vi "generate_pulse.vi"() -> ()   [LabVIEW 2018]
uses:
  Control 1.ctl
  <vilib>/DAQmx/write.llb/DAQmx Write (Analog 1D Wfm NChan NSamp).vi
  <vilib>/DAQmx/create/channels.llb/DAQmx Create Channel (AO-Voltage-Basic).vi
  <vilib>/DAQmx/configure/timing.llb/DAQmx Timing (Sample Clock).vi
  <vilib>/DAQmx/miscellaneous.llb/DAQmx Fill In Error Info.vi
  <resource>/objmgr/daqmx.rc
panel:
  in  "Exit":bool
  out "Actual Sample Rate 2":dbl=400000.0 format="%0.2f"
  in  "Physical Channel(s)":tag="Dev3/ao0:1"
  in  "Min Voltage 2":dbl=-10.0
  in  "Max Voltage 2":dbl=10.0
  in  "Sample Clock Source":tag="OnboardClock"
  in  "Sample Rate 2":dbl=400000.0 format="%#_6p"
  in  "Pulser Cycles":i32=10
  out "Sample per Channel AO":dbl=20000.0
  in  "Tab Control 4":enum32{"Basic", "Gaussian", "Chirp"}(tab)=enum."Chirp"
  in  "Pulse Basic":T2={"Basic amp"=1.5, "Duty cycle %"=50.0, "Basic freq (Hz)"=200, "Basic Type"=2} {"Basic Type" items=["Sine Wave", "Triangle Wave", "Square Wave", "Sawtooth Wave"]; "Duty cycle %" format="%#.2f"; "Basic amp" format="%0.2p"}
  in  "Pulse Gaussian":T3={"Gauss amp"=2.8, "Gauss Nor. Band"=0.5, "Gauss atten (dB)"=6.0, "Gauss freq (Hz)"=1000.0}
  in  "Pulse chirp":T4={"Chirp amp"=2.1, "Chirp f2"=1500.0, "Chirp f1"=500.0} {"Chirp f1" format="%0.2f"; "Chirp f2" format="%0.2f"; "Chirp amp" format="%0.2f"}
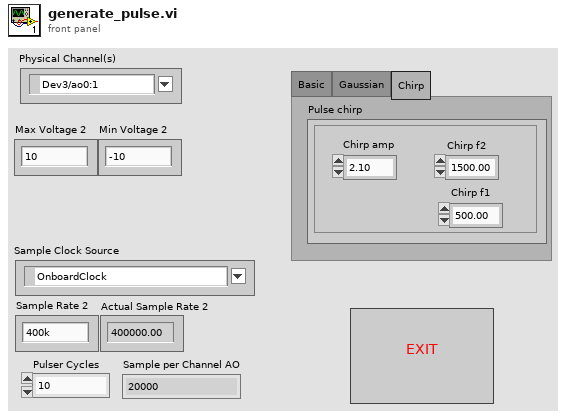
[diagram p1: front panel]
types:
  T1 = typedef "Control 1.ctl" = dbl
  T2 = cluster{"Basic amp":T1, "Duty cycle %":dbl, "Basic freq (Hz)":u16, "Basic Type":u16}
  T3 = cluster{"Gauss amp":dbl, "Gauss Nor. Band":dbl, "Gauss atten (dB)":dbl, "Gauss freq (Hz)":dbl}
  T4 = cluster{"Chirp amp":dbl, "Chirp f2":dbl, "Chirp f1":dbl}
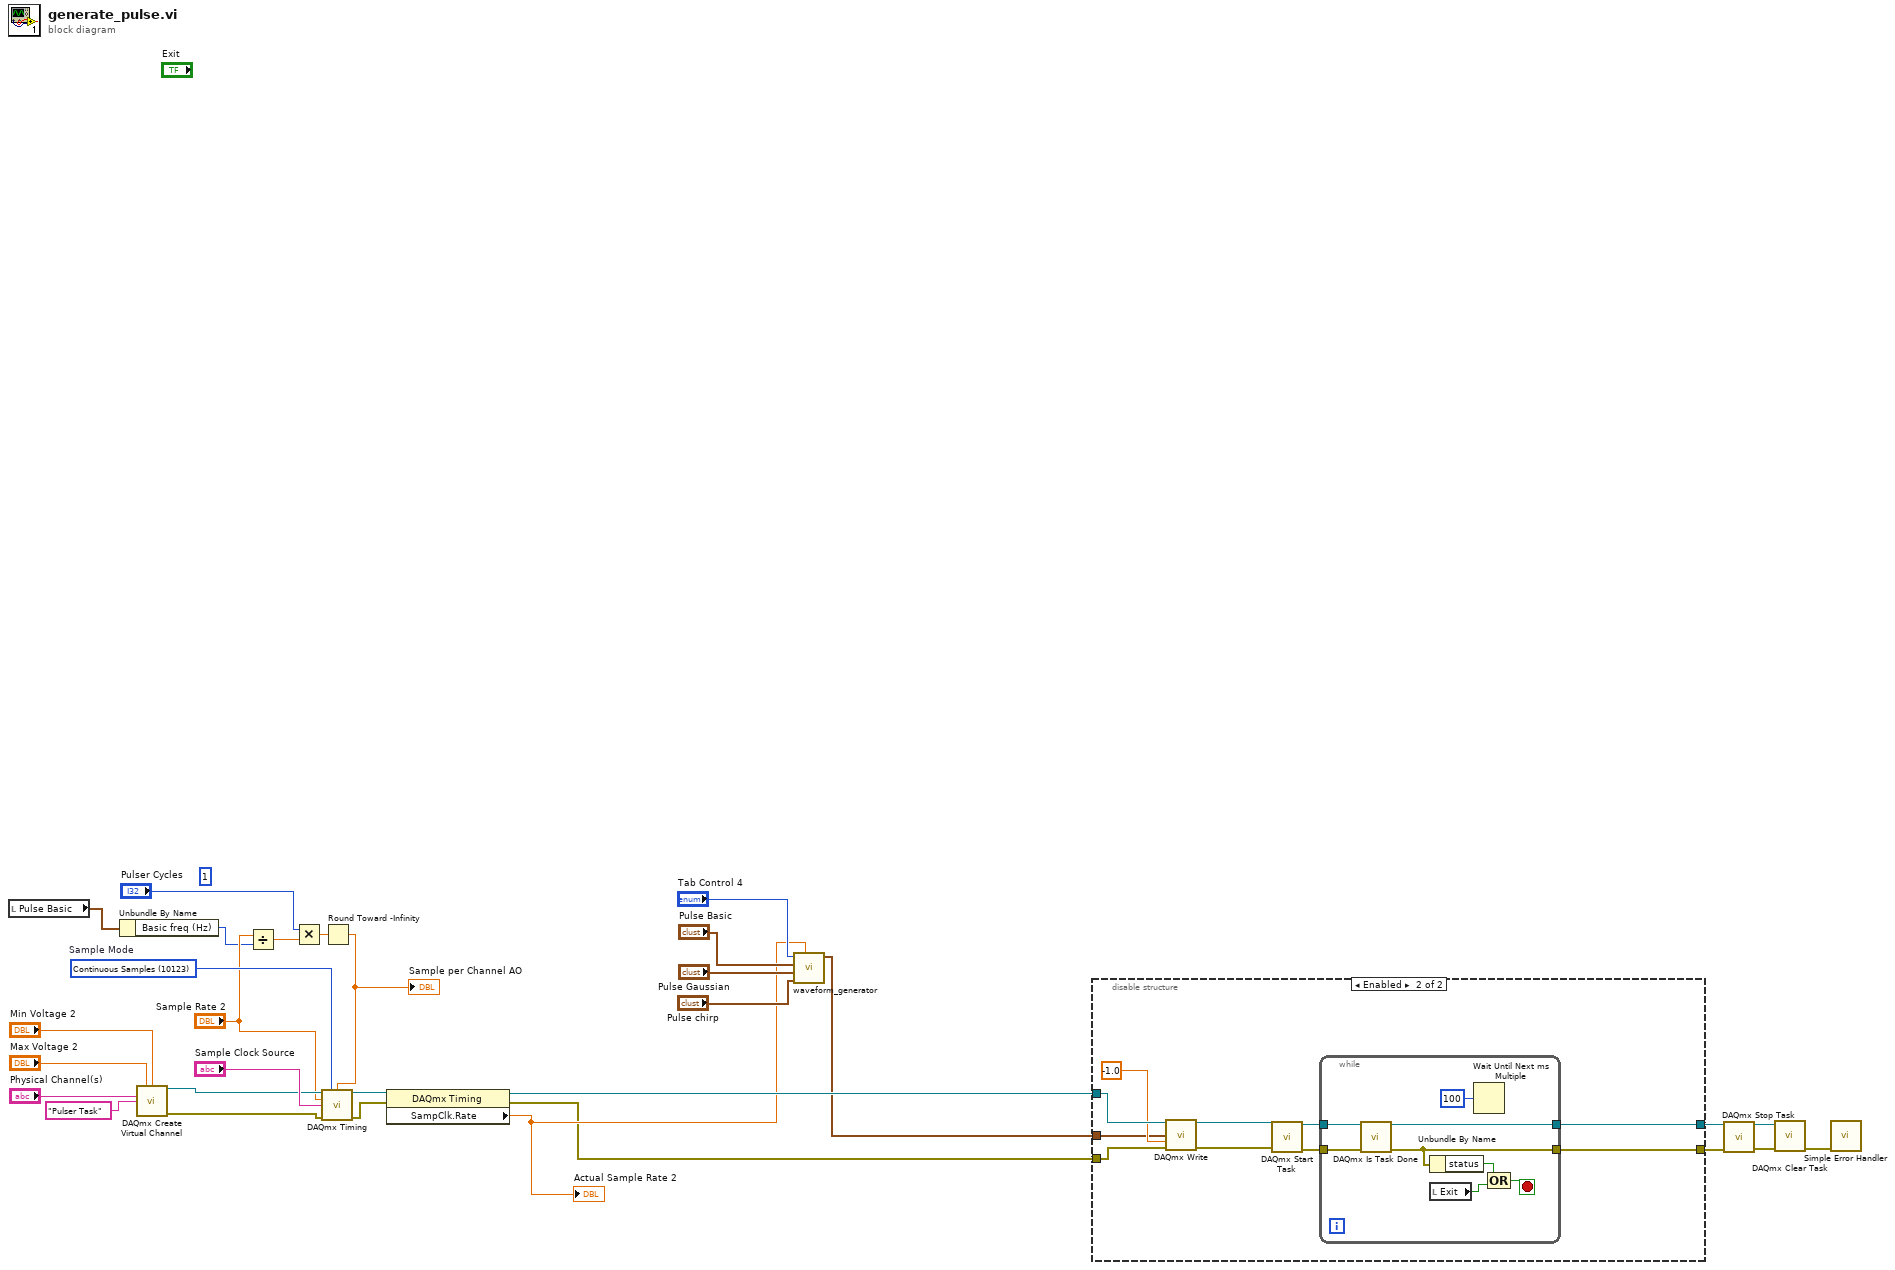
[diagram p0: block diagram]
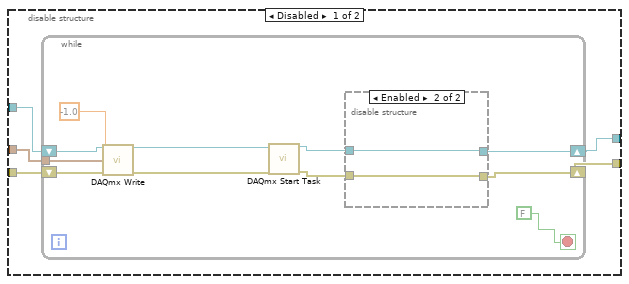
[diagram p2: hidden frame]
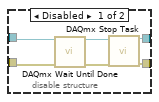
[diagram p3: hidden frame]
diagram:
  (unwired) 1 ("x")
  w28 = 10123 items=["Finite Samples"=10178, "Continuous Samples"=10123, "Hardware Timed Single Point"=12522]  # Sample Mode
  n1 = local read "Pulse Basic"() -> (w2:T2)
  n2 = Unbundle By Name(w2) -> ("Basic freq (Hz)"=w1:u16)
  n3 = call-poly <vilib>:"DAQmx Create Virtual Channel.vi"("maximum value"="Max Voltage 2", "minimum value"="Min Voltage 2", "physical channels"="Physical Channel(s)", "name to assign"="Pulser Task") -> ("task out"=w22:refnum<k21>, "error out"=w21:errorcluster)  [unwired: 10 in]
  n4 = Divide(x="Sample Rate 2", y=w1) -> (x/y=w19:dbl)
  n5 = Multiply(x="Pulser Cycles", y=w19) -> (x*y=w18:dbl)
  n6 = Round Toward -Infinity(1:w18) -> (0:w10:dbl)
  "Sample per Channel AO" <- w10
  n7 = call-poly <vilib>:"DAQmx Timing.vi"("task/channels in"=w22, "sample mode"=w28, "samples per channel"=w10, "rate"="Sample Rate 2", "source"="Sample Clock Source", "error in"=w21) -> ("task out"=w30:refnum<k21>, "error out"=w29:errorcluster)  [unwired: 8 in]
  n8 = property class="DAQmx Timing"(reference=w30, error in=w29) -> (reference out=w17:refnum<k21>, error out=w3:errorcluster, "SampClk.Rate"=w5:dbl)
  "Actual Sample Rate 2" <- w5
  n9 = call "waveform_generator.vi"("Sampling rate"=w5, "Pulse chirp"="Pulse chirp", "Pulse Gaussian"="Pulse Gaussian", "Cluster Basic"="Pulse Basic", "Tab Control"="Tab Control 4") -> ("Waveform Graph"=w4:waveform(dbl)[])  [unwired: 6 in]
  n10 = disable-structure shown="Enabled" {
    disable-tunnel: w4 -> [w35 w56]
    disable-tunnel: [w34 w59] -> w14
    disable-tunnel: [w33 w58] -> w11
    disable-tunnel: w17 -> [w32 w60]
    disable-tunnel: w3 -> [w31 w55]
    frame Disabled {
      n11 = while {
        tunnel: w35 -> [w46]
        shift-right: [w42] -> w34
        shift-left: w32 -> [w40]
        shift-right: [w41] -> w33
        shift-left: w31 -> [w39]
        stop <- FALSE stop-if-true
        n12 = call-poly <vilib>:"DAQmx Write.vi"("task/channels in"=w40, "data"=w46, "timeout"=-1.0, "error in"=w39) -> ("task out"=w45:refnum<k21>, "error out"=w44:errorcluster)  [unwired: 9 in, 1 out]
        n13 = call <vilib>:"DAQmx Start Task.vi"("task/channels in"=w45, "error in"=w44) -> ("task out"=w38:refnum<k21>, "error out"=w37:errorcluster)  [unwired: 12 in]
        n14 = disable-structure shown="Enabled" {
          disable-tunnel: [w52 w54] -> w42
          disable-tunnel: [w51 w53] -> w41
          disable-tunnel: w38 -> [w50 w54]
          disable-tunnel: w37 -> [w49 w53]
          frame Disabled {
            n15 = call <vilib>:"DAQmx Wait Until Done.vi"("task/channels in"=w50, "error in"=w49) -> ("task out"=w48:refnum<k21>, "error out"=w47:errorcluster)  [unwired: 12 in]
            n16 = call <vilib>:"DAQmx Stop Task.vi"("task/channels in"=w48, "error in"=w47) -> ("task out"=w52:refnum<k21>, "error out"=w51:errorcluster)  [unwired: 12 in]
          }
          frame Enabled {
          }
        }
      }
    }
    frame Enabled {
      n17 = call-poly <vilib>:"DAQmx Write.vi"("task/channels in"=w60, "data"=w56, "timeout"=-1.0, "error in"=w55) -> ("task out"=w62:refnum<k21>, "error out"=w64:errorcluster)  [unwired: 9 in, 1 out]
      n18 = call <vilib>:"DAQmx Start Task.vi"("task/channels in"=w62, "error in"=w64) -> ("task out"=w61:refnum<k21>, "error out"=w63:errorcluster)  [unwired: 12 in]
      n19 = while {
        tunnel: w61 -> [w72]
        tunnel: w63 -> [w71]
        tunnel: [w69] -> w58
        tunnel: [w70] -> w59
        stop <- w66 stop-if-true
        n20 = call <vilib>:"DAQmx Is Task Done.vi"("task/channels in"=w72, "error in"=w71) -> ("task out"=w70:refnum<k21>, "error out"=w69:errorcluster)  [unwired: 11 in, 1 out]
        n21 = Unbundle By Name(w69) -> ("status"=w67:bool)
        n22 = local read "Exit"() -> (w65:bool)
        n23 = Wait Until Next ms Multiple(millisecond multiple=u32 100) -> ()  [unwired: 1 out]
        n24 = Compound Arithmetic op=OR(w67, w65) -> (w66:bool)
      }
    }
  }
  n25 = call <vilib>:"DAQmx Stop Task.vi"("task/channels in"=w14, "error in"=w11) -> ("task out"=w13:refnum<k21>, "error out"=w12:errorcluster)  [unwired: 12 in]
  n26 = call <vilib>:"DAQmx Clear Task.vi"("task in"=w13, "error in"=w12) -> ("error out"=w27:errorcluster)  [unwired: 13 in]
  n27 = call <vilib>:"Simple Error Handler.vi"("error in (no error)"=w27) -> ()  [unwired: 4 in, 5 out]
